vi "And.vi"(0 "X":i32, 5 "Y":i32, 11 "Error_In":errorcluster) -> (4 "Output":i32, 15 "Error_Out":errorcluster)   [LabVIEW 2023]
doc: "Perform AND operation"
uses:
  Controls/Notifier_Operation_Select.ctl
panel:
  # "AND"
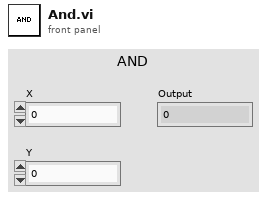
[diagram p1: front panel]
types:
  T1 = typedef "Notifier_Operation_Select.ctl" = enum16{"Obtain_Notifier", "Send_Notification", "Get_Notification_Status", "Release_Notifier"}
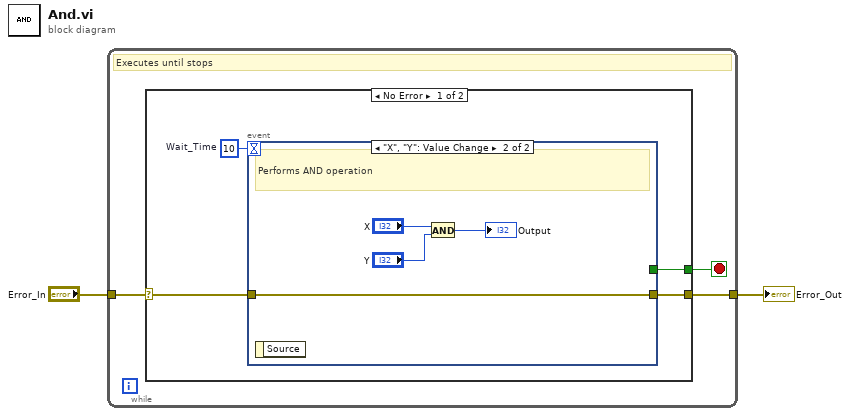
[diagram p0: block diagram]
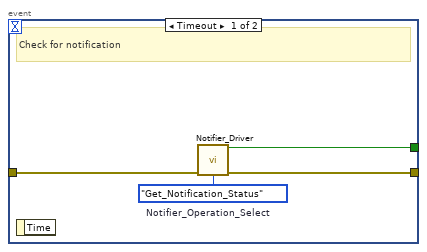
[diagram p2: hidden frame]
diagram:
  n1 = while {
    tunnel: "Error_In" -> [w3]
    tunnel: [w5] -> w1
    stop <- w4 stop-if-true
    # "Executes until stops"
    n2 = case shown="No Error" w3 {
      selector: w3 -> [w7 w18]
      tunnel: [w9 w18] -> w5
      tunnel: [w8 _] -> w4
      frame No Error {
        w6 = 10  # Wait_Time
        n3 = event shown="[1] \"X\", \"Y\": Value Change" {
          selector: _ -> [_ _]
          dyn-events: _ -> [_ _]
          timeout: w6 -> [_ _]
          tunnel: w7 -> [w13 w17]
          tunnel: [w12 w17] -> w9
          tunnel: [w10 _] -> w8
          event Timeout {
            w11 = Notifier_Operation_Select."Get_Notification_Status"  # Notifier_Operation_Select
            # "Check for notification"
            n4 = event-data() -> ()  [unwired: 1 in, 1 out]
            n5 = call "Notifier_Driver.vi"("Error_In"=w13, "Notifier_Operation_Select"=w11) -> ("Latest_Notification"=w10:bool, "Error_Out"=w12:errorcluster)  [unwired: 12 in]
          }
          event "X", "Y": Value Change {
            # "Performs AND operation"
            n6 = event-data() -> ()  [unwired: 1 in, 1 out]
            n7 = And(x="X", y="Y") -> (x .and. y?=→"Output":i32)
          }
        }
      }
      frame Error {
      }
    }
  }
  "Error_Out" <- w1
